vi "CRYSet Post Processing Front Panel.vi"(11 "Vi Ref":refnum<vi>) -> ()   [LabVIEW 2013]
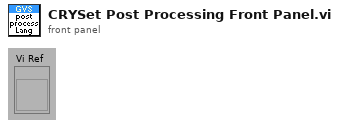
[diagram p1: front panel]
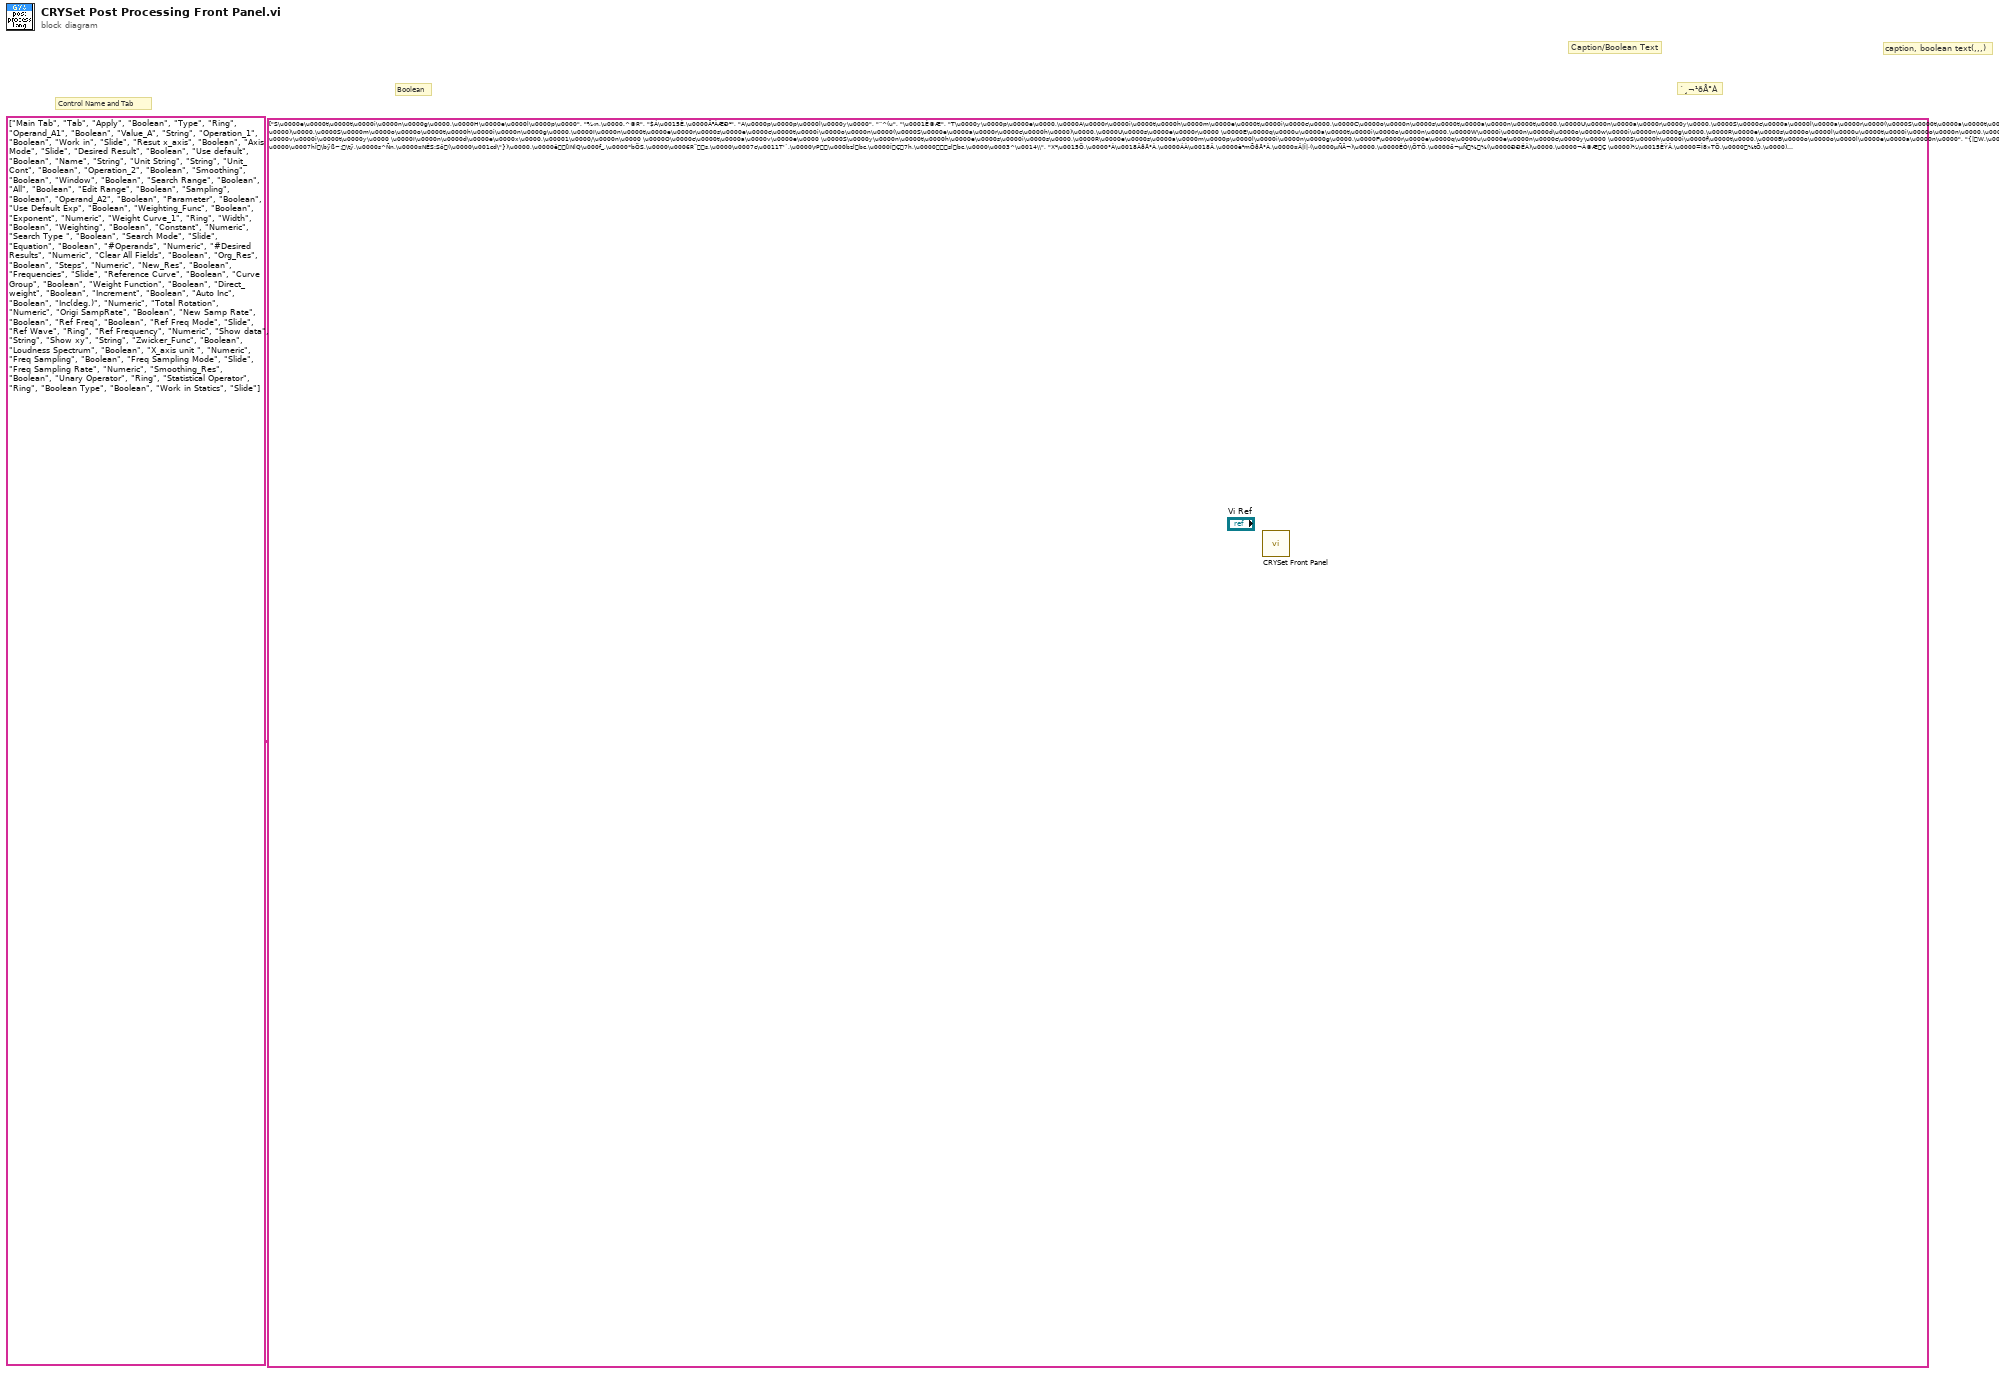
[diagram p0: block diagram]
diagram:
  # "`¸¬¹ðÅ°À"
  # "Boolean"
  # "Caption, Tab Page, Multilist Header, Button 4"
  # "Control Type"
  # "Control Name and Tab"
  # "caption, boolean text(,,,)"
  # "Caption/Boolean Text"
  n1 = call "CRYSet Front Panel.vi"("Caption(Boolean Text)"=string[][] [["S\u0000e\u0000t\u0000t\u0000i\u0000n\u0000g\u0000,\u0000H\u0000e\u0000l\u0000p\u0000", "¾‹n,\u0000.^©R", "$Á\u0015È,\u0000Ä³ÀÆÐ¹"], ["A\u0000p\u0000p\u0000l\u0000y\u0000", "”^(u", "\u0001È©Æ"], ["T\u0000y\u0000p\u0000e\u0000,\u0000A\u0000r\u0000i\u0000t\u0000h\u0000m\u0000e\u0000t\u0000i\u0000c\u0000,\u0000C\u0000o\u0000n\u0000s\u0000t\u0000a\u0000n\u0000t\u0000,\u0000U\u0000n\u0000a\u0000r\u0000y\u0000,\u0000S\u0000c\u0000a\u0000l\u0000a\u0000r\u0000(\u0000S\u0000t\u0000a\u0000t\u0000i\u0000s\u0000t\u0000i\u0000c\u0000s\u0000)\u0000,\u0000S\u0000m\u0000o\u0000o\u0000t\u0000h\u0000i\u0000n\u0000g\u0000,\u0000I\u0000n\u0000t\u0000e\u0000r\u0000s\u0000e\u0000c\u0000t\u0000i\u0000o\u0000n\u0000(\u0000S\u0000e\u0000a\u0000r\u0000c\u0000h\u0000)\u0000,\u0000U\u0000s\u0000e\u0000r\u0000 \u0000E\u0000q\u0000u\u0000a\u0000t\u0000i\u0000o\u0000n\u0000,\u0000W\u0000i\u0000n\u0000d\u0000o\u0000w\u0000i\u0000n\u0000g\u0000,\u0000R\u0000e\u0000s\u0000o\u0000l\u0000u\u0000t\u0000i\u0000o\u0000n\u0000,\u0000D\u0000i\u0000r\u0000e\u0000c\u0000t\u0000i\u0000v\u0000i\u0000t\u0000y\u0000 \u0000I\u0000n\u0000d\u0000e\u0000x\u0000,\u00001\u0000/\u0000n\u0000 \u0000O\u0000c\u0000t\u0000a\u0000v\u0000e\u0000 \u0000S\u0000y\u0000n\u0000t\u0000h\u0000e\u0000s\u0000i\u0000s\u0000,\u0000R\u0000e\u0000s\u0000a\u0000m\u0000p\u0000l\u0000i\u0000n\u0000g\u0000,\u0000F\u0000r\u0000e\u0000q\u0000u\u0000e\u0000n\u0000c\u0000y\u0000 \u0000S\u0000h\u0000i\u0000f\u0000t\u0000,\u0000B\u0000o\u0000o\u0000l\u0000e\u0000a\u0000n\u0000", "{|W,\u0000{peÐ{,\u00008^pe,\u0000\u0000NCQÐ{,\u0000\u0007hÏ\bÿß~¡\tÿ,\u0000s^Ñn,\u0000¤NÉS:Sô(\u0000\u001cd\"})\u0000,\u0000ê[INlQ\u000f_,\u0000*bÖS,\u0000\u0006R¨s,\u0000\u0007c\u0011T'`,\u0000\rP\u000bzlbc,\u0000ÍÇ7h,\u0000slbc,\u0000\u0003^\u0014\\", "X¹\u0015Ö,\u0000°À\u0018ÂðÅ°À,\u0000ÁÀ\u0018Â,\u0000è²mÕðÅ°À,\u0000¤Â|Î|·(\u0000µÑÄ¬)\u0000,\u0000ÉÓ\\ÖTÖ,\u0000õ¬µÑ½½(\u0000ÐÐÉÀ)\u0000,\u0000¬À©ÆÇ \u0000)¼\u0015ÈÝÂ,\u0000=Ì8»TÖ,\u0000½tÕ,\u0000)¼¥Õ¨Ì\u0018Â,\u00001\u0000/\u0000n\u0000%ÆÀÐ\f¾iÕ1Á,\u0000¬Ç\\Ôø¼TÖ,\u0000üÈ\fÓ\u0018Â.Æ@®,\u0000`¸¬¹ðÅ°À"], ["O\u0000p\u0000e\u0000r\u0000a\u0000n\u0000d\u0000 \u0000A\u0000", "Íd\\Ope \u0000A\u0000", "ðÅ°À\u0018Â \u0000A\u0000"], ["V\u0000a\u0000l\u0000u\u0000e\u0000", "<P", "\u0012¬"], ["O\u0000p\u0000e\u0000r\u0000a\u0000t\u0000i\u0000o\u0000n\u0000", "Ð{", "ðÅ°À"], ["W\u0000o\u0000r\u0000k\u0000 \u0000i\u0000n\u0000,\u0000d\u0000B\u0000,\u0000L\u0000i\u0000n\u0000e\u0000a\u0000r\u0000,\u0000P\u0000o\u0000w\u0000e\u0000r\u0000", "Ð{!j\u000f_,\u0000\u0006R\u001d(\u0000d\u0000B\u0000)\u0000,\u0000¿~'`,\u0000Rs", "ðÅ°À)¼ÝÂ,\u0000\\¸ø­,\u0000 Á\u0015Ö,\u0000\u001cÈñ¬"], ["R\u0000e\u0000s\u0000u\u0000l\u0000t\u0000 \u0000x\u0000-\u0000a\u0000x\u0000i\u0000s\u0000 \u0000s\u0000a\u0000m\u0000e\u0000 \u0000a\u0000s\u0000:\u0000", "Ó~gX\u0000t", "°¬ü¬X\u0000•Í"], ["A\u0000x\u0000i\u0000s\u0000 \u0000M\u0000o\u0000d\u0000e\u0000,\u0000O\u0000p\u0000e\u0000r\u0000a\u0000n\u0000d\u0000 \u0000A\u0000,\u0000O\u0000p\u0000e\u0000r\u0000a\u0000n\u0000d\u0000 \u0000B\u0000,\u0000A\u0000 \u0000&\u0000 \u0000B\u0000 \u0000c\u0000o\u0000m\u0000b\u0000i\u0000n\u0000e\u0000d\u0000", "A\u0000x\u0000i\u0000s\u0000 \u0000M\u0000o\u0000d\u0000e\u0000,\u0000Íd\\OpeA\u0000,\u0000Íd\\OpeB\u0000,\u0000A\u0000ŒTB\u0000Ó~\bT", "A\u0000x\u0000i\u0000s\u0000 \u0000M\u0000o\u0000d\u0000e\u0000,\u0000ðÅ°À\u0018Â \u0000A\u0000,\u0000ðÅ°À\u0018Â \u0000B\u0000,\u0000A\u0000@ÆB\u0000XÇ \u0000°¬iÕ"], ["D\u0000e\u0000s\u0000i\u0000r\u0000e\u0000d\u0000 \u0000R\u0000e\u0000s\u0000u\u0000l\u0000t\u0000", "Ó~œg", "\u0014¼|·”² \u0000°¬ü¬"], ["U\u0000s\u0000e\u0000 \u0000d\u0000e\u0000f\u0000a\u0000u\u0000l\u0000t\u0000", "O(uØž¤‹<P", "0®\u0015È\u0012¬ \u0000¬¹©Æ"], ["N\u0000a\u0000m\u0000e\u0000", "\rTðy", "tÇ„¹"], ["U\u0000n\u0000i\u0000t\u0000", "USMO", "è²\u0004Ç"], ["U\u0000n\u0000i\u0000t\u0000.\u0000.\u0000.\u0000", "USMO", "è²\u0004Ç"], ["O\u0000p\u0000e\u0000r\u0000a\u0000t\u0000i\u0000o\u0000n\u0000", "Ð{", "ðÅ°À"], ["S\u0000m\u0000o\u0000o\u0000t\u0000h\u0000i\u0000n\u0000g\u0000 \u0000W\u0000i\u0000d\u0000t\u0000h\u0000(\u0000H\u0000z\u0000)\u0000", "s^Ñn½[¦^(\u0000H\u0000z\u0000)\u0000", "ÉÓ\\Ö\b±D¾(\u0000H\u0000z\u0000)\u0000"], ["W\u0000i\u0000n\u0000d\u0000o\u0000w\u0000", "—zãS", "=ÌhÕ\u0018Â"], ["S\u0000e\u0000a\u0000r\u0000c\u0000h\u0000 \u0000R\u0000a\u0000n\u0000g\u0000e\u0000", "\u001cd\"}\u0003ƒôV", "ÐÐÉÀ”¼\u0004Ç"], ["A\u0000l\u0000l\u0000", "@b\tg", "\u0004È´Ì"], ["E\u0000d\u0000i\u0000t\u0000 \u0000R\u0000a\u0000n\u0000g\u0000e\u0000.\u0000.\u0000.\u0000", "\u0016\u0003ôV", "”¼\u0004Ç¸ÓÑÉ"], ["S\u0000a\u0000m\u0000p\u0000l\u0000i\u0000n\u0000g\u0000 \u0000R\u0000a\u0000t\u0000e\u0000", "Ç‘7h‡s", "\\Ôø¼TÖ`¹"], ["O\u0000p\u0000e\u0000r\u0000a\u0000n\u0000d\u0000 \u0000A\u0000", "Íd\\Ope \u0000A\u0000", "ðÅ°À\u0018Â \u0000A\u0000"], ["P\u0000a\u0000r\u0000a\u0000m\u0000e\u0000t\u0000e\u0000r\u0000s\u0000", "ÂSpe", "À¼\u0018Â"], ["U\u0000s\u0000e\u0000 \u0000D\u0000e\u0000f\u0000a\u0000u\u0000l\u0000t\u0000 \u0000V\u0000a\u0000l\u0000u\u0000e\u0000s\u0000", "(u7bØž¤‹<P", "0®\u0015È\u0012¬ \u0000¬¹©Æ"], ["W\u0000e\u0000i\u0000g\u0000h\u0000t\u0000i\u0000n\u0000g\u0000 \u0000F\u0000u\u0000n\u0000c\u0000t\u0000i\u0000o\u0000n\u0000", " RCgýQpe", "4»Œ¬hÕ\u0018Â"], ["E\u0000x\u0000p\u0000o\u0000n\u0000e\u0000n\u0000t\u0000", "\u0007cpe", "ÀÉ\u0018Â"], ["W\u0000e\u0000i\u0000g\u0000h\u0000t\u0000i\u0000n\u0000g\u0000 \u0000C\u0000u\u0000r\u0000v\u0000e\u0000", " RCgòf¿~", "4»Œ¬á¬ Á"], ["W\u0000i\u0000d\u0000t\u0000h\u0000", "½[¦^", "\b±D¾"], ["W\u0000e\u0000i\u0000g\u0000h\u0000t\u0000i\u0000n\u0000g\u0000", " RCg", "4»Œ¬"], ["C\u0000o\u0000n\u0000s\u0000t\u0000a\u0000n\u0000t\u0000", "8^pe", "ÁÀ\u0018Â"], ["S\u0000e\u0000a\u0000r\u0000c\u0000h\u0000 \u0000T\u0000y\u0000p\u0000e\u0000 ", "\u001cd\"}{|‹W", "ÐÐÉÀX¹\u0015Ö"], ["S\u0000e\u0000a\u0000r\u0000c\u0000h\u0000 \u0000M\u0000o\u0000d\u0000e\u0000,\u0000S\u0000e\u0000a\u0000r\u0000c\u0000h\u0000 \u0000U\u0000p\u0000,\u0000S\u0000e\u0000a\u0000r\u0000c\u0000h\u0000 \u0000D\u0000o\u0000w\u0000n\u0000,\u0000R\u0000e\u0000t\u0000u\u0000r\u0000n\u0000 \u0000a\u0000l\u0000l\u0000 \u0000i\u0000n\u0000t\u0000e\u0000r\u0000s\u0000e\u0000c\u0000t\u0000i\u0000o\u0000n\u0000 \u0000p\u0000o\u0000i\u0000n\u0000t\u0000s\u0000", "S\u0000e\u0000a\u0000r\u0000c\u0000h\u0000 \u0000M\u0000o\u0000d\u0000e\u0000,\u0000\u0011T\nN\u001cd\"},\u0000\u0011T\u000bN\u001cd\"},\u0000ÔÞV@b\tgv¤N¹p", "S\u0000e\u0000a\u0000r\u0000c\u0000h\u0000 \u0000M\u0000o\u0000d\u0000e\u0000,\u0000ÃÆ)¼¥Õ \u0000 \u0000ÐÐÉÀ,\u0000DÅ˜·)¼¥Õ \u0000 \u0000ÐÐÉÀ,\u0000\u0004È´Ì \u0000¬ÀÐ­\u0010È"], ["E\u0000q\u0000u\u0000a\u0000t\u0000i\u0000o\u0000n\u0000 \u0000(\u0000e\u0000.\u0000g\u0000.\u0000 \u0000x\u0000=\u0000a\u00000\u0000+\u0000a\u00001\u0000;\u0000)\u0000", "lQ\u000f_ \u0000(\u0000e\u0000.\u0000g\u0000.\u0000 \u0000x\u0000=\u0000a\u00000\u0000+\u0000a\u00001\u0000;\u0000)\u0000", ")¼\u0015ÈÝÂ \u0000(\u0000e\u0000.\u0000g\u0000.\u0000 \u0000x\u0000=\u0000a\u00000\u0000+\u0000a\u00001\u0000;\u0000)\u0000"], ["#\u0000 \u0000o\u0000f\u0000 \u0000O\u0000p\u0000e\u0000r\u0000a\u0000n\u0000d\u0000s\u0000", "Íd\\Ope*Npe", "ðÅ°À\u0018Â\u001c¬\u0018Â"], ["#\u0000 \u0000o\u0000f\u0000 \u0000D\u0000e\u0000s\u0000i\u0000r\u0000e\u0000d\u0000 \u0000R\u0000e\u0000s\u0000u\u0000l\u0000t\u0000s\u0000", "Ó~œg*Npe", "\u0014¼|·”² \u0000°¬ü¬\u001c¬\u0018Â"], ["C\u0000l\u0000e\u0000a\u0000r\u0000 \u0000A\u0000l\u0000l\u0000 \u0000F\u0000i\u0000e\u0000l\u0000d\u0000s\u0000", "\u0005nd–@b\tg„v†˜ßW", "¨ºà´ \u00009¸íÅ­À\u001cÈ"], ["O\u0000r\u0000i\u0000g\u0000i\u0000n\u0000a\u0000l\u0000 \u0000R\u0000e\u0000s\u0000o\u0000l\u0000u\u0000t\u0000i\u0000o\u0000n\u0000", "SËY\u0006R¨s", "\bÍ0®„½tÕ`¹"], ["S\u0000t\u0000e\u0000p\u0000s\u0000", "ek¤š", "x¬LÇ"], ["N\u0000e\u0000w\u0000 \u0000R\u0000e\u0000s\u0000o\u0000l\u0000u\u0000t\u0000i\u0000o\u0000n\u0000", "°ev\u0006R¨s", "ÈÀ \u0000„½tÕ`¹"], ["F\u0000r\u0000e\u0000q\u0000u\u0000e\u0000n\u0000c\u0000i\u0000e\u0000s\u0000,\u0000I\u0000S\u0000O\u0000,\u0000R\u0000T\u0000A\u0000", "‘˜‡s,\u0000I\u0000S\u0000O\u0000,\u0000R\u0000T\u0000A\u0000", "üÈ\fÓ\u0018Â,\u0000I\u0000S\u0000O\u0000,\u0000R\u0000T\u0000A\u0000"], ["R\u0000e\u0000f\u0000e\u0000r\u0000e\u0000n\u0000c\u0000e\u0000 \u0000C\u0000u\u0000r\u0000v\u0000e\u0000", "ÂS\u0003€òf¿~", "8Ìà¬á¬ Á"], ["C\u0000u\u0000r\u0000v\u0000e\u0000 \u0000G\u0000r\u0000o\u0000u\u0000p\u0000", "òf¿~Ä~", "á¬ ÁqÈ"], ["W\u0000e\u0000i\u0000g\u0000h\u0000t\u0000i\u0000n\u0000g\u0000 \u0000F\u0000u\u0000n\u0000c\u0000t\u0000i\u0000o\u0000n\u0000", " RCgýQpe", "4»Œ¬hÕ\u0018Â"], ["W\u0000e\u0000i\u0000g\u0000h\u0000t\u0000i\u0000n\u0000g\u0000", " RCg", "4»Œ¬"], ["I\u0000n\u0000c\u0000r\u0000e\u0000m\u0000e\u0000n\u0000t\u0000a\u0000t\u0000i\u0000o\u0000n\u0000", "žXÏ‘", "É\u0000¬É·"], ["A\u0000u\u0000t\u0000o\u0000 \u0000I\u0000n\u0000c\u0000r\u0000e\u0000m\u0000e\u0000n\u0000t\u0000", "ê¨RXÏ", "ÇÙ³É\u0000¬"], ["I\u0000n\u0000c\u0000(\u0000d\u0000e\u0000g\u0000.\u0000)\u0000", "žXÏ‘(\u0000d\u0000e\u0000g\u0000.\u0000)\u0000", "É\u0000¬É·(\u0000d\u0000e\u0000g\u0000.\u0000)\u0000"], ["T\u0000o\u0000t\u0000a\u0000l\u0000 \u0000R\u0000o\u0000t\u0000a\u0000t\u0000i\u0000o\u0000n\u0000", ";`Ëel", "\u001dÍŒÖ\u0004È"], ["O\u0000r\u0000i\u0000g\u0000i\u0000n\u0000a\u0000l\u0000 \u0000S\u0000a\u0000m\u0000p\u0000l\u0000i\u0000n\u0000g\u0000 \u0000R\u0000a\u0000t\u0000e\u0000", "ŸSËYÇ‘7h‡s", "\bÍ0®\\Ôø¼TÖ`¹"], ["N\u0000e\u0000w\u0000 \u0000S\u0000a\u0000m\u0000p\u0000l\u0000i\u0000n\u0000g\u0000 \u0000R\u0000a\u0000t\u0000e\u0000", "°eÇ‘7h‡s", "ÈÀ \u0000\\Ôø¼TÖ`¹"], ["R\u0000e\u0000f\u0000e\u0000r\u0000e\u0000n\u0000c\u0000e\u0000 \u0000F\u0000r\u0000e\u0000q\u0000u\u0000e\u0000n\u0000c\u0000y\u0000", "ÂS\u0003€‘˜‡s", "8Ìà¬üÈ\fÓ\u0018Â"], ["R\u0000e\u0000f\u0000 \u0000F\u0000r\u0000e\u0000q\u0000 \u0000M\u0000o\u0000d\u0000e\u0000,\u0000A\u0000u\u0000t\u0000o\u0000m\u0000a\u0000t\u0000i\u0000c\u0000,\u0000U\u0000s\u0000e\u0000r\u0000 \u0000D\u0000e\u0000f\u0000i\u0000n\u0000e\u0000d\u0000", "R\u0000e\u0000f\u0000 \u0000F\u0000r\u0000e\u0000q\u0000 \u0000M\u0000o\u0000d\u0000e\u0000,\u0000ê¨R,\u0000(u7b[IN", "R\u0000e\u0000f\u0000 \u0000F\u0000r\u0000e\u0000q\u0000 \u0000M\u0000o\u0000d\u0000e\u0000,\u0000ÇÙ³,\u0000¬À©ÆÇ\u0015ÈXÇ"], ["R\u0000e\u0000f\u0000e\u0000r\u0000e\u0000n\u0000c\u0000e\u0000 \u0000W\u0000a\u0000v\u0000e\u0000f\u0000o\u0000r\u0000m\u0000", "ÂS\u0003€âlb_", "8Ìà¬\fÓ\u0015Ö"], ["R\u0000e\u0000f\u0000e\u0000r\u0000e\u0000n\u0000c\u0000e\u0000 \u0000F\u0000r\u0000e\u0000q\u0000u\u0000e\u0000n\u0000c\u0000y\u0000", "ÂS\u0003€‘˜‡s", "8Ìà¬üÈ\fÓ\u0018Â"], ["S\u0000h\u0000o\u0000w\u0000 \u0000d\u0000a\u0000t\u0000a\u0000,\u0000S\u0000h\u0000o\u0000w\u0000 \u0000D\u0000a\u0000t\u0000a\u0000", "S\u0000h\u0000o\u0000w\u0000 \u0000d\u0000a\u0000t\u0000a\u0000,\u0000>f:ypenc", "S\u0000h\u0000o\u0000w\u0000 \u0000d\u0000a\u0000t\u0000a\u0000,\u0000ÇÌ¸ô¼0®"], ["S\u0000h\u0000o\u0000w\u0000 \u0000x\u0000y\u0000,\u0000S\u0000h\u0000o\u0000w\u0000 \u0000D\u0000a\u0000t\u0000a\u0000", "S\u0000h\u0000o\u0000w\u0000 \u0000x\u0000y\u0000,\u0000>f:ypenc", "S\u0000h\u0000o\u0000w\u0000 \u0000x\u0000y\u0000,\u0000ÇÌ¸ô¼0®"], ["Z\u0000w\u0000i\u0000c\u0000k\u0000e\u0000r\u0000", "Z\u0000w\u0000i\u0000c\u0000k\u0000e\u0000r\u0000", "Z\u0000w\u0000i\u0000c\u0000k\u0000e\u0000r\u0000"], ["L\u0000o\u0000u\u0000d\u0000n\u0000e\u0000s\u0000s\u0000 \u0000S\u0000p\u0000e\u0000c\u0000t\u0000r\u0000u\u0000m\u0000", "IQ1Œ", "¤Â™Ó¸Òü·"], ["X\u0000_\u0000a\u0000x\u0000i\u0000s\u0000 \u0000u\u0000n\u0000i\u0000t\u0000 \u0000", "X\u0000tUSMO", "X\u0000•Íè²\u0004Ç"], ["P\u0000l\u0000a\u0000y\u0000b\u0000a\u0000c\u0000k\u0000 \u0000S\u0000a\u0000m\u0000p\u0000l\u0000i\u0000n\u0000g\u0000 \u0000R\u0000a\u0000t\u0000e\u0000", "‘˜‡s", "¬ÇÝÀ\\Ôø¼TÖ`¹"], ["F\u0000r\u0000e\u0000q\u0000 \u0000S\u0000a\u0000m\u0000p\u0000l\u0000i\u0000n\u0000g\u0000 \u0000M\u0000o\u0000d\u0000e\u0000,\u0000A\u0000u\u0000t\u0000o\u0000m\u0000a\u0000t\u0000i\u0000c\u0000a\u0000l\u0000l\u0000y\u0000 \u0000C\u0000a\u0000l\u0000c\u0000u\u0000l\u0000a\u0000t\u0000e\u0000d\u0000,\u0000U\u0000s\u0000e\u0000r\u0000 \u0000D\u0000e\u0000f\u0000i\u0000n\u0000e\u0000d\u0000", "F\u0000r\u0000e\u0000q\u0000 \u0000S\u0000a\u0000m\u0000p\u0000l\u0000i\u0000n\u0000g\u0000 \u0000M\u0000o\u0000d\u0000e\u0000,\u0000ꁨR,\u0000ꁚ[IN", "F\u0000r\u0000e\u0000q\u0000 \u0000S\u0000a\u0000m\u0000p\u0000l\u0000i\u0000n\u0000g\u0000 \u0000M\u0000o\u0000d\u0000e\u0000,\u0000ÇÙ³Ä¬°À,\u0000¬¹©ÆÇ\u0015ÈXÇ"], ["P\u0000l\u0000a\u0000y\u0000b\u0000a\u0000c\u0000k\u0000 \u0000S\u0000a\u0000m\u0000p\u0000l\u0000i\u0000n\u0000g\u0000 \u0000R\u0000a\u0000t\u0000e\u0000", "‘˜‡s", "¬ÇÝÀ\\Ôø¼TÖ`¹"], ["S\u0000m\u0000o\u0000o\u0000t\u0000h\u0000i\u0000n\u0000g\u0000", "s^Ñn", "ÉÓ\\Ö"], ["U\u0000n\u0000a\u0000r\u0000y\u0000 \u0000O\u0000p\u0000e\u0000r\u0000a\u0000t\u0000o\u0000r\u0000,\u0000C\u0000h\u0000a\u0000n\u0000g\u0000e\u0000 \u0000S\u0000i\u0000g\u0000n\u0000,\u0000R\u0000e\u0000c\u0000i\u0000p\u0000r\u0000o\u0000c\u0000a\u0000l\u0000 \u0000V\u0000a\u0000l\u0000u\u0000e\u0000,\u0000A\u0000b\u0000s\u0000o\u0000l\u0000u\u0000t\u0000e\u0000 \u0000V\u0000a\u0000l\u0000u\u0000e\u0000,\u0000S\u0000q\u0000u\u0000a\u0000r\u0000e\u0000,\u0000S\u0000q\u0000u\u0000a\u0000r\u0000e\u0000 \u0000R\u0000o\u0000o\u0000t\u0000,\u0000E\u0000x\u0000p\u0000,\u0000L\u0000n\u0000,\u0000U\u0000n\u0000w\u0000r\u0000a\u0000p\u0000 \u0000P\u0000h\u0000a\u0000s\u0000e\u0000,\u0000G\u0000r\u0000o\u0000u\u0000p\u0000 \u0000D\u0000e\u0000l\u0000a\u0000y\u0000,\u0000F\u0000F\u0000T\u0000,\u0000I\u0000n\u0000v\u0000e\u0000r\u0000s\u0000e\u0000 \u0000F\u0000F\u0000T\u0000", "U\u0000n\u0000a\u0000r\u0000y\u0000 \u0000O\u0000p\u0000e\u0000r\u0000a\u0000t\u0000o\u0000r\u0000,\u0000øvÍSpe,\u0000\u0012Ppe,\u0000Ý~ù[<P,\u0000s^¹e,\u0000s^¹e9h,\u0000\u0007cpe,\u0000ê6qù[pe,\u0000U\u0000n\u0000w\u0000r\u0000a\u0000p\u0000 \u0000P\u0000h\u0000a\u0000s\u0000e\u0000,\u0000G\u0000r\u0000o\u0000u\u0000p\u0000 \u0000D\u0000e\u0000l\u0000a\u0000y\u0000,\u0000F\u0000F\u0000T\u0000,\u0000I\u0000n\u0000v\u0000e\u0000r\u0000s\u0000e\u0000 \u0000F\u0000F\u0000T\u0000", "U\u0000n\u0000a\u0000r\u0000y\u0000 \u0000O\u0000p\u0000e\u0000r\u0000a\u0000t\u0000o\u0000r\u0000,\u0000C\u0000h\u0000a\u0000n\u0000g\u0000e\u0000 \u0000S\u0000i\u0000g\u0000n\u0000,\u0000R\u0000e\u0000c\u0000i\u0000p\u0000r\u0000o\u0000c\u0000a\u0000l\u0000 \u0000V\u0000a\u0000l\u0000u\u0000e\u0000,\u0000A\u0000b\u0000s\u0000o\u0000l\u0000u\u0000t\u0000e\u0000 \u0000V\u0000a\u0000l\u0000u\u0000e\u0000,\u0000S\u0000q\u0000u\u0000a\u0000r\u0000e\u0000,\u0000S\u0000q\u0000u\u0000a\u0000r\u0000e\u0000 \u0000R\u0000o\u0000o\u0000t\u0000,\u0000E\u0000x\u0000p\u0000,\u0000L\u0000n\u0000,\u0000U\u0000n\u0000w\u0000r\u0000a\u0000p\u0000 \u0000P\u0000h\u0000a\u0000s\u0000e\u0000,\u0000G\u0000r\u0000o\u0000u\u0000p\u0000 \u0000D\u0000e\u0000l\u0000a\u0000y\u0000,\u0000F\u0000F\u0000T\u0000,\u0000I\u0000n\u0000v\u0000e\u0000r\u0000s\u0000e\u0000 \u0000F\u0000F\u0000T\u0000"], ["S\u0000t\u0000a\u0000t\u0000i\u0000s\u0000t\u0000i\u0000c\u0000a\u0000l\u0000 \u0000O\u0000p\u0000e\u0000r\u0000a\u0000t\u0000o\u0000r\u0000,\u0000A\u0000v\u0000e\u0000r\u0000a\u0000g\u0000e\u0000,\u0000P\u0000o\u0000w\u0000e\u0000r\u0000 \u0000S\u0000u\u0000m\u0000,\u0000M\u0000a\u0000x\u0000i\u0000m\u0000u\u0000m\u0000,\u0000M\u0000i\u0000n\u0000i\u0000m\u0000u\u0000m\u0000,\u0000E\u0000s\u0000t\u0000.\u0000 \u0000R\u0000e\u0000s\u0000o\u0000n\u0000a\u0000n\u0000c\u0000e\u0000,\u0000E\u0000s\u0000t\u0000.\u0000 \u0000N\u0000o\u0000t\u0000c\u0000h\u0000,\u0000I\u0000E\u0000E\u0000E\u0000 \u0000T\u0000O\u0000L\u0000R\u0000,\u0000I\u0000E\u0000E\u0000E\u0000 \u0000R\u0000O\u0000L\u0000R\u0000,\u0000I\u0000E\u0000E\u0000E\u0000 \u0000S\u0000O\u0000L\u0000R\u0000,\u0000I\u0000T\u0000U\u0000-\u0000T\u0000 \u0000S\u0000L\u0000R\u0000,\u0000I\u0000T\u0000U\u0000-\u0000T\u0000 \u0000R\u0000L\u0000R\u0000,\u0000I\u0000T\u0000U\u0000-\u0000T\u0000 \u0000R\u0000L\u0000R\u0000 \u0000w\u0000/\u0000 \u0000L\u0000e\u0000a\u0000k\u0000,\u0000I\u0000T\u0000U\u0000-\u0000T\u0000 \u0000S\u0000T\u0000M\u0000R\u0000,\u0000A\u0000t\u0000t\u0000a\u0000c\u0000k\u0000 \u0000T\u0000i\u0000m\u0000e\u0000,\u0000R\u0000e\u0000l\u0000e\u0000a\u0000s\u0000e\u0000 \u0000T\u0000i\u0000m\u0000e\u0000,\u0000Z\u0000w\u0000i\u0000c\u0000k\u0000e\u0000r\u0000 \u0000L\u0000o\u0000u\u0000d\u0000n\u0000e\u0000s\u0000s\u0000", "S\u0000t\u0000a\u0000t\u0000i\u0000s\u0000t\u0000i\u0000c\u0000a\u0000l\u0000 \u0000O\u0000p\u0000e\u0000r\u0000a\u0000t\u0000o\u0000r\u0000,\u0000s^GW<P,\u0000ŸR‡s;`ŒT,\u0000\u0000g'Y<P,\u0000\u0000g\u000f\\<P,\u0000\u0010Œ/c0O—{,\u0000ÍS\u0010Œ/c0O—{,\u0000I\u0000E\u0000E\u0000E\u0000 \u0000T\u0000O\u0000L\u0000R\u0000,\u0000I\u0000E\u0000E\u0000E\u0000 \u0000R\u0000O\u0000L\u0000R\u0000,\u0000I\u0000E\u0000E\u0000E\u0000 \u0000S\u0000O\u0000L\u0000R\u0000,\u0000I\u0000T\u0000U\u0000-\u0000T\u0000 \u0000S\u0000L\u0000R\u0000,\u0000I\u0000T\u0000U\u0000-\u0000T\u0000 \u0000R\u0000L\u0000R\u0000,\u0000I\u0000T\u0000U\u0000-\u0000T\u0000 \u0000R\u0000L\u0000R\u0000 \u0000w\u0000/\u0000 \u0000L\u0000e\u0000a\u0000k\u0000,\u0000I\u0000T\u0000U\u0000-\u0000T\u0000 \u0000S\u0000T\u0000M\u0000R\u0000,\u0000A\u0000t\u0000t\u0000a\u0000c\u0000k\u0000 \u0000T\u0000i\u0000m\u0000e\u0000,\u0000R\u0000e\u0000l\u0000e\u0000a\u0000s\u0000e\u0000 \u0000T\u0000i\u0000m\u0000e\u0000,\u0000Z\u0000w\u0000i\u0000c\u0000k\u0000e\u0000r\u0000 \u0000L\u0000o\u0000u\u0000d\u0000n\u0000e\u0000s\u0000s\u0000", "S\u0000t\u0000a\u0000t\u0000i\u0000s\u0000t\u0000i\u0000c\u0000a\u0000l\u0000 \u0000O\u0000p\u0000e\u0000r\u0000a\u0000t\u0000o\u0000r\u0000,\u0000A\u0000v\u0000e\u0000r\u0000a\u0000g\u0000e\u0000,\u0000P\u0000o\u0000w\u0000e\u0000r\u0000 \u0000S\u0000u\u0000m\u0000,\u0000M\u0000a\u0000x\u0000i\u0000m\u0000u\u0000m\u0000,\u0000M\u0000i\u0000n\u0000i\u0000m\u0000u\u0000m\u0000,\u0000E\u0000s\u0000t\u0000.\u0000 \u0000R\u0000e\u0000s\u0000o\u0000n\u0000a\u0000n\u0000c\u0000e\u0000,\u0000E\u0000s\u0000t\u0000.\u0000 \u0000N\u0000o\u0000t\u0000c\u0000h\u0000,\u0000I\u0000E\u0000E\u0000E\u0000 \u0000T\u0000O\u0000L\u0000R\u0000,\u0000I\u0000E\u0000E\u0000E\u0000 \u0000R\u0000O\u0000L\u0000R\u0000,\u0000I\u0000E\u0000E\u0000E\u0000 \u0000S\u0000O\u0000L\u0000R\u0000,\u0000I\u0000T\u0000U\u0000-\u0000T\u0000 \u0000S\u0000L\u0000R\u0000,\u0000I\u0000T\u0000U\u0000-\u0000T\u0000 \u0000R\u0000L\u0000R\u0000,\u0000I\u0000T\u0000U\u0000-\u0000T\u0000 \u0000R\u0000L\u0000R\u0000 \u0000w\u0000/\u0000 \u0000L\u0000e\u0000a\u0000k\u0000,\u0000I\u0000T\u0000U\u0000-\u0000T\u0000 \u0000S\u0000T\u0000M\u0000R\u0000,\u0000A\u0000t\u0000t\u0000a\u0000c\u0000k\u0000 \u0000T\u0000i\u0000m\u0000e\u0000,\u0000R\u0000e\u0000l\u0000e\u0000a\u0000s\u0000e\u0000 \u0000T\u0000i\u0000m\u0000e\u0000,\u0000Z\u0000w\u0000i\u0000c\u0000k\u0000e\u0000r\u0000 \u0000L\u0000o\u0000u\u0000d\u0000n\u0000e\u0000s\u0000s\u0000"], ["R\u0000e\u0000s\u0000u\u0000l\u0000t\u0000", "Ó~œg", "°¬ü¬\u0012¬"], ["W\u0000o\u0000r\u0000k\u0000 \u0000i\u0000n\u0000,\u0000d\u0000B\u0000,\u0000L\u0000i\u0000n\u0000e\u0000a\u0000r\u0000,\u0000P\u0000o\u0000w\u0000e\u0000r\u0000", "Ð{!j\u000f_,\u0000\u0006R\u001d(\u0000d\u0000B\u0000)\u0000,\u0000¿~'`,\u0000Rs", "ðÅ°À)¼ÝÂ,\u0000\\¸ø­,\u0000 Á\u0015Ö,\u0000\u001cÈñ¬"]], "Control ID and Type(Label Name, Type)"=string[][] [["Main Tab", "Tab"], ["Apply", "Boolean"], ["Type", "Ring"], ["Operand_A1", "Boolean"], ["Value_A", "String"], ["Operation_1", "Boolean"], ["Work in", "Slide"], ["Resut x_axis", "Boolean"], ["Axis Mode", "Slide"], ["Desired Result", "Boolean"], ["Use default", "Boolean"], ["Name", "String"], ["Unit String", "String"], ["Unit_Cont", "Boolean"], ["Operation_2", "Boolean"], ["Smoothing", "Boolean"], ["Window", "Boolean"], ["Search Range", "Boolean"], ["All", "Boolean"], ["Edit Range", "Boolean"], ["Sampling", "Boolean"], ["Operand_A2", "Boolean"], ["Parameter", "Boolean"], ["Use Default Exp", "Boolean"], ["Weighting_Func", "Boolean"], ["Exponent", "Numeric"], ["Weight Curve_1", "Ring"], ["Width", "Boolean"], ["Weighting", "Boolean"], ["Constant", "Numeric"], ["Search Type ", "Boolean"], ["Search Mode", "Slide"], ["Equation", "Boolean"], ["#Operands", "Numeric"], ["#Desired Results", "Numeric"], ["Clear All Fields", "Boolean"], ["Org_Res", "Boolean"], ["Steps", "Numeric"], ["New_Res", "Boolean"], ["Frequencies", "Slide"], ["Reference Curve", "Boolean"], ["Curve Group", "Boolean"], ["Weight Function", "Boolean"], ["Direct_weight", "Boolean"], ["Increment", "Boolean"], ["Auto Inc", "Boolean"], ["Inc(deg.)", "Numeric"], ["Total Rotation", "Numeric"], ["Origi SampRate", "Boolean"], ["New Samp Rate", "Boolean"], ["Ref Freq", "Boolean"], ["Ref Freq Mode", "Slide"], ["Ref Wave", "Ring"], ["Ref Frequency", "Numeric"], ["Show data", "String"], ["Show xy", "String"], ["Zwicker_Func", "Boolean"], ["Loudness Spectrum", "Boolean"], ["X_axis unit ", "Numeric"], ["Freq Sampling", "Boolean"], ["Freq Sampling Mode", "Slide"], ["Freq Sampling Rate", "Numeric"], ["Smoothing_Res", "Boolean"], ["Unary Operator", "Ring"], ["Statistical Operator", "Ring"], ["Boolean Type", "Boolean"], ["Work in Statics", "Slide"]], "Vi Ref"="Vi Ref") -> ()  [unwired: 9 in]
